vi "Driver Init.vi"(8 "error in (no error)":errorcluster, 11 "AD4212C in":refnum<class "AD4212C.lvclass">) -> (0 "error out":errorcluster, 3 "AD4212C out":refnum<class "AD4212C.lvclass">)   [LabVIEW 2014, in "AD4212C.lvlib" / "AD4212C.lvclass"]
doc: "Inicializa el Valor del puerto COM con un valor seteado en código y puesto como variable. (Este valor varia según el puerto y la pc al cual se conecte el dispositivo)."
uses:
  AD4212C.lvclass
  AD4212C.lvclass/AD4212C.ctl
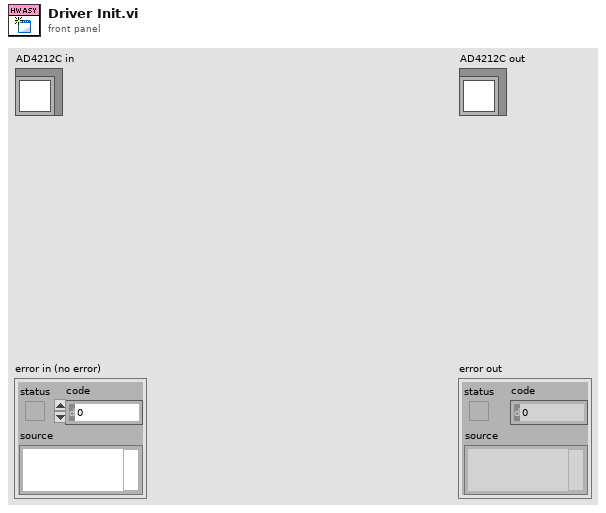
[diagram p1: front panel]
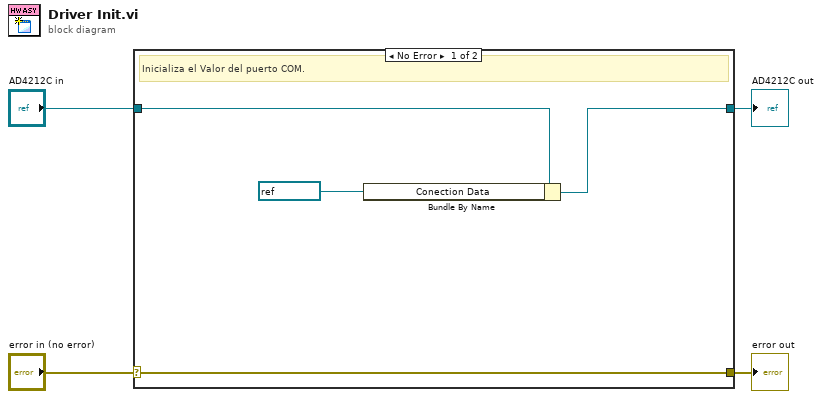
[diagram p0: block diagram]
diagram:
  n1 = case shown="No Error" "error in (no error)" {
    selector: "error in (no error)" -> [w8 w10]
    tunnel: [w8 w10] -> w3
    tunnel: [w6 w9] -> w1
    tunnel: "AD4212C in" -> [w7 w9]
    frame No Error {
      # "Inicializa el Valor del puerto COM."
      n2 = Bundle By Name(cluster=w7, "Conection Data"=refnum<visa-resource-name> "COM4" ("Conection Data.VISA resource name")) -> (w6:refnum<class "AD4212C.lvclass">)
    }
    frame Error {
    }
  }
  "error out" <- w3
  "AD4212C out" <- w1
